vi "Encrypt Letter (objdict).vi"(8 "error in (no error)":errorcluster, 10 "letter":string, 11 "objdict in":refnum<class "objdict.lvclass">) -> (0 "error out":errorcluster, 2 "encrypted letter":string, 3 "objdict out":refnum<class "objdict.lvclass">)   [LabVIEW 2015]
uses:
  objdict/objdict.lvclass
  Letter/Letter.lvclass
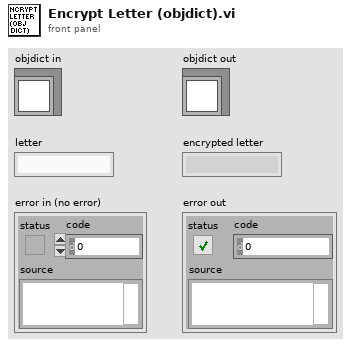
[diagram p1: front panel]
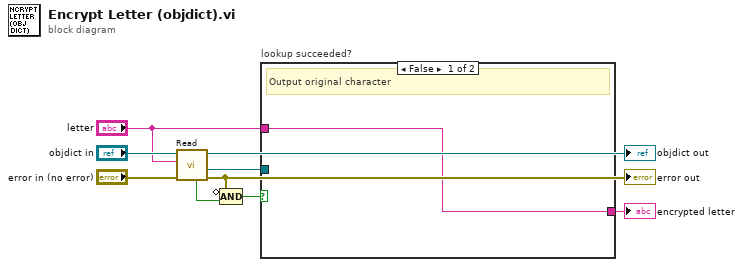
[diagram p0: block diagram]
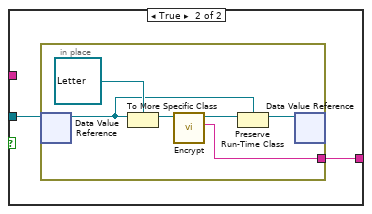
[diagram p2: hidden frame]
diagram:
  n1 = call "Read.vi"("error in (no error)"="error in (no error)", "key"="letter", "Object Dictionary in"="objdict in") -> ("error out"=w8:errorcluster, "Object ref"=w9:refnum<data-value>, "Object Dictionary out"=→"objdict out":refnum<class "objdict.lvclass">, "found"=w6:bool)  [unwired: 5 in]
  "error out" <- w8
  n2 = Compound Arithmetic op=AND(invert w8, w6) -> (w7:bool)
  n3 = case "lookup succeeded?" shown="False" w7 {
    tunnel: w9 -> [_ w12]
    tunnel: [w10 w11] -> w2
    tunnel: "letter" -> [w10 _]
    frame False {
      # "Output original character"
    }
    frame True {
      n4 = in-place {
        in-place-border: [w13] -> w11
        n5 = in-place-dvr #1(w12) -> (w17:refnum<class>)  [unwired: 1 out]
        n6 = To More Specific Class(target class=refnum<class "Letter.lvclass"> refnum ("Letter.lvclass"), reference=w17) -> (specific class reference=w15:refnum<class "Letter.lvclass">)  [unwired: 1 in, 1 out]
        n7 = call "Encrypt.vi"("Letter in"=w15) -> ("letter"=w13:string, "Letter out"=w14:refnum<class "Letter.lvclass">)  [unwired: 9 in]
        n8 = Preserve Run-Time Class(object in=w14, 2:w17) -> (object out=w16:refnum<class>)  [unwired: 1 in, 1 out]
        n9 = in-place-dvr #1(w16) -> ()  [unwired: 2 out]
      }
    }
  }
  "encrypted letter" <- w2
